vi "PI Database Check.vi"(8 "error in (no error)":errorcluster, 10 "PI Fields":T6[](array[typedef]), 11 "PI Test Parameters In":T1={"Measurement"={"sxFieldId"="", "sValue"="", "nDataType"=enum."Scalar", "sUnits"="", "sDisplayName"=""}, "Limit"={"Limits On"=TRUE, "Limits"=[]}}) -> (0 "error out":errorcluster, 3 "PI Test Parameters Out":T1={"Measurement"={"sxFieldId"="", "sValue"="", "nDataType"=enum."Scalar", "sUnits"="", "sDisplayName"=""}, "Limit"={"Limits On"=TRUE, "Limits"=[]}})   [LabVIEW 2011]
uses:
  server/database/Fields/Field Record.ctl
  server/database/Fields/Field DataTypes.ctl
  server/database/Fields/Field NextItem.ctl
  TypeDefs/PI Test Parameters.ctl
  TypeDefs/PI Measurement Cluster.ctl
  TypeDefs/PI Limit Parameters.ctl
  TypeDefs/PI Limit Definition.ctl
  TypeDefs/PI Limit Comparison.ctl
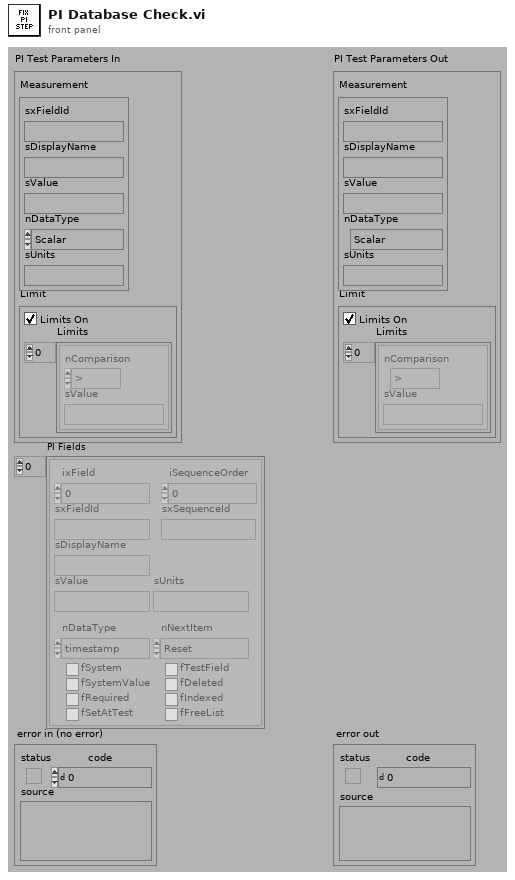
[diagram p1: front panel]
types:
  T1 = typedef "PI Test Parameters.ctl" = cluster{"Measurement":T2, "Limit":T3}
  T2 = typedef "PI Measurement Cluster.ctl" = cluster{"sxFieldId":string, "sValue":string, "nDataType":enum16{"Scalar", "Enumeration"}, "sUnits":string, "sDisplayName":string}
  T3 = typedef "PI Limit Parameters.ctl" = cluster{"Limits On":bool, "Limits":T4[]}
  T4 = typedef "PI Limit Definition.ctl" = cluster{"nComparison":T5, "sValue":string}
  T5 = typedef "PI Limit Comparison.ctl" = enum16{">", ">=", "<", "<=", "<>", "="}
  T6 = typedef "Field Record.ctl" = cluster{"ixField":i32, "iSequenceOrder":i32, "sxFieldId":string, "sxSequenceId":string, "sDisplayName":string, "sValue":string, "sUnits":string, "nDataType":T7, "nNextItem":T8, "fSystem":bool, "fSystemValue":bool, "fRequired":bool, "fSetAtTest":bool, "fTestField":bool, "fDeleted":bool, "fIndexed":bool, "fFreeList":bool}
  T7 = typedef "Field DataTypes.ctl" = enum32{"text", "numeric", "list", "timestamp", "boolean"}
  T8 = typedef "Field NextItem.ctl" = enum32{"Reset", "Retain", "Auto-Increment"}
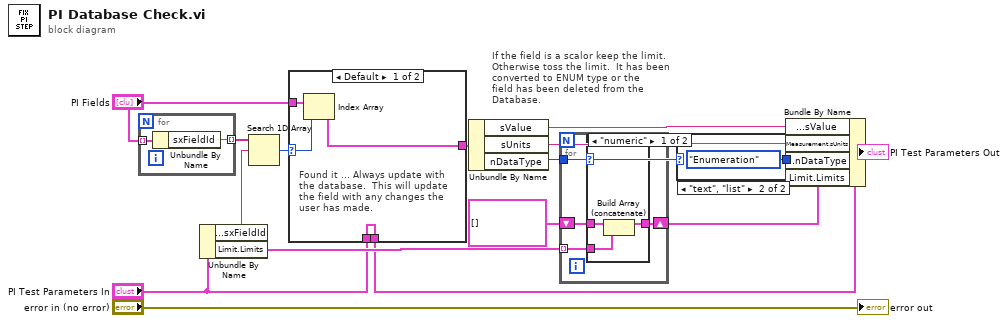
[diagram p0: block diagram]
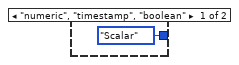
[diagram p2: hidden frame]
diagram:
  # "If the field is a scalor keep the limit.\nOtherwise toss the limit.  It has been\nconverted to ENUM type or the\nfield has been deleted from the \nDatabase."
  n1 = for {
    tunnel: "PI Fields" -> [w18] mode=indexing
    tunnel: [w17] -> w15 mode=indexing
    n2 = Unbundle By Name(w18) -> ("sxFieldId"=w17:string)
  }
  n3 = Unbundle By Name("PI Test Parameters In") -> ("Measurement.sxFieldId"=w9:string, "Limit.Limits"=w13:T4[])
  n4 = Search 1D Array(1D array=w15, element=w9) -> (index of element=w10:i32)  [unwired: 1 out]
  n5 = case shown="Default" w10 {
    selector: w10 -> [w21 _]
    tunnel: "PI Fields" -> [w22 _]
    tunnel: [w20 _] -> w5
    tunnel: "PI Test Parameters In" -> [w19 _]
    tunnel: [w19 _] -> w8
    frame Default {
      # "Found it ... Always update with\nthe database.  This will update\nthe field with any changes the\nuser has made."
      n6 = Index Array(array=w22, index=w21) -> (element=w20:T6)
    }
    frame -1 {
      # "This PI was not found\nremove from the PI\nmeasurement."
    }
  }
  n7 = Unbundle By Name(w5) -> ("sValue"=w3:string, "sUnits"=w4:string, "nDataType"=w2:T7)
  n8 = for {
    tunnel: w13 -> [w24] mode=indexing
    shift-right: [w25] -> w12
    shift-left: T4[] [] -> [w26]
    tunnel: w2 -> [w23]
    n9 = case shown="\"numeric\"" w23 {
      tunnel: w26 -> [w29 w30]
      tunnel: [w27 w30] -> w25
      tunnel: w24 -> [w28 _]
      frame "numeric" {
        n10 = Build Array (concatenate)(w29, w28) -> (w27:T4[])
      }
      frame "text", "list".."boolean" {
      }
    }
  }
  n11 = case shown="\"text\", \"list\"" w2 {
    tunnel: [enum16{"Scalar", "Enumeration"}."Scalar" ("Measurement.Type") enum16{"Scalar", "Enumeration"}."Enumeration" ("Measurement.Type")] -> w1
    frame "numeric", "timestamp", "boolean" {
    }
    frame "text", "list" {
    }
  }
  n12 = Bundle By Name(cluster=w8, "Measurement.sValue"=w3, "Measurement.sUnits"=w4, "Measurement.nDataType"=w1, "Limit.Limits"=w12) -> (→"PI Test Parameters Out":T1)
  "error out" <- "error in (no error)"
